vi "Bitfile.Unload.vi"(11 "Session":u32) -> ()   [LabVIEW 2019, in "Diagnostics Addon Engine.lvlib"]
uses:
  Diagnostics Addon Engine.lvlib
  NiFpga.dll
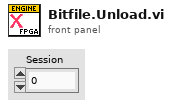
[diagram p1: front panel]
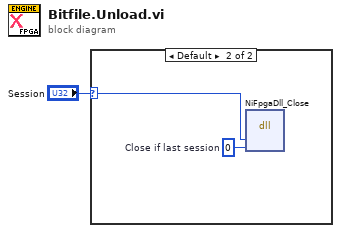
[diagram p0: block diagram]
diagram:
  n1 = case shown="Default" "Session" {
    selector: "Session" -> [_ w2]
    frame 0 {
    }
    frame Default {
      w3 = u32 0  # Close if last session
      n2 = dll-call lib="NiFpga.dll" fn="NiFpgaDll_Close"("Session"=w2, "Attribute"=w3) -> ()  [unwired: 6 in, 2 out]
    }
  }
